vi "Voigt_Fit_DLL_Test.vi"() -> ()   [LabVIEW 2020]
doc: "Test the operation of the Lorentzian Model Fit DLL inside LabVIEW\n\nThe code should do the following\n1. read in a data file containing measured LLM data [freq (MHz), spctrm (dBm)]\n1a. select a subset of the data from some subset of the freq range (optional)\n2. provide initial guesses for the fitting parameters\n3. call the function Lorentz_Fit from the DLL\n\nR. Sheehan 9 - 11 - 2021"
uses:
  <vilib>/Utility/file.llb/Read Delimited Spreadsheet (DBL).vi
panel:
  out "Lor_gof":dbl[](array[numeric])=[3199.0, 1.0009386733416772, 0.954874518705434, 0.4817149539059473]
  out "L_pars":dbl[](array[numeric])=[0.7072584069399376, 80.0, 1.7560129064005117]
  out "Voigt LLM / MHz":dbl
  in  "Freqs":T1={"Ffitlo / MHz"=70.0, "Fcentre / MHz"=80.0, "Ffithi / MHz"=90.0, "Lor HWHM / MHz"=2.6187499999999915, "Peak Est / nW"=0.0, "Gau stdev / MHz "=2.6187499999999915}
  in  "Fcentre / MHz":dbl=80.0
  out "gof_stats":dbl[](array[numeric])=[4799.0, 1.000625521267723, 0.9428903903200956, 0.4850704566774246]
  out "V_pars":dbl[](array[numeric])=[2.3238013033110674, 80.0, 1.3781481716459836]
  out "FileName":path=path "C:/Users/robertsheehan/Programming/LabVIEW/Textronix_RSA2203A/Sample_Data/Smpl_LLM_1.txt"
  in  "Ffithi / MHz":dbl=95.0
  in  "Ffitlo / MHz":dbl=65.0
  out "Fmax / MHz":dbl=80.19375
  out "LLest / MHz":dbl=2.299999999999997
  out "Pmax / nW":dbl=1.4094510581310635e-06
  out "Pmax / dBm":dbl=-58.5095
  out "Flo / MHz":dbl=60.0
  out "Fhi / MHz":dbl=100.0
  out "LLM Output":cluster{"all rows":dbl[], "all rows":dbl[]}[](graph)
  out "TheData":dbl[][](array[numeric])
  # "Amp. Par\n\nAOM Freq / MHz\n\nLor HWHM / MHz\n\nGau Stdev / MHz"
  # "Amp. Par\n\nAOM Freq / MHz\n\nLor HWHM / MHz"
  # "chi^{2} for the fit\n\nchi^{2} / nu\n\nR^{2}\n\nGOF"
  # "chi^{2} for the fit\n\nchi^{2} / nu\n\nR^{2}\n\nGOF"
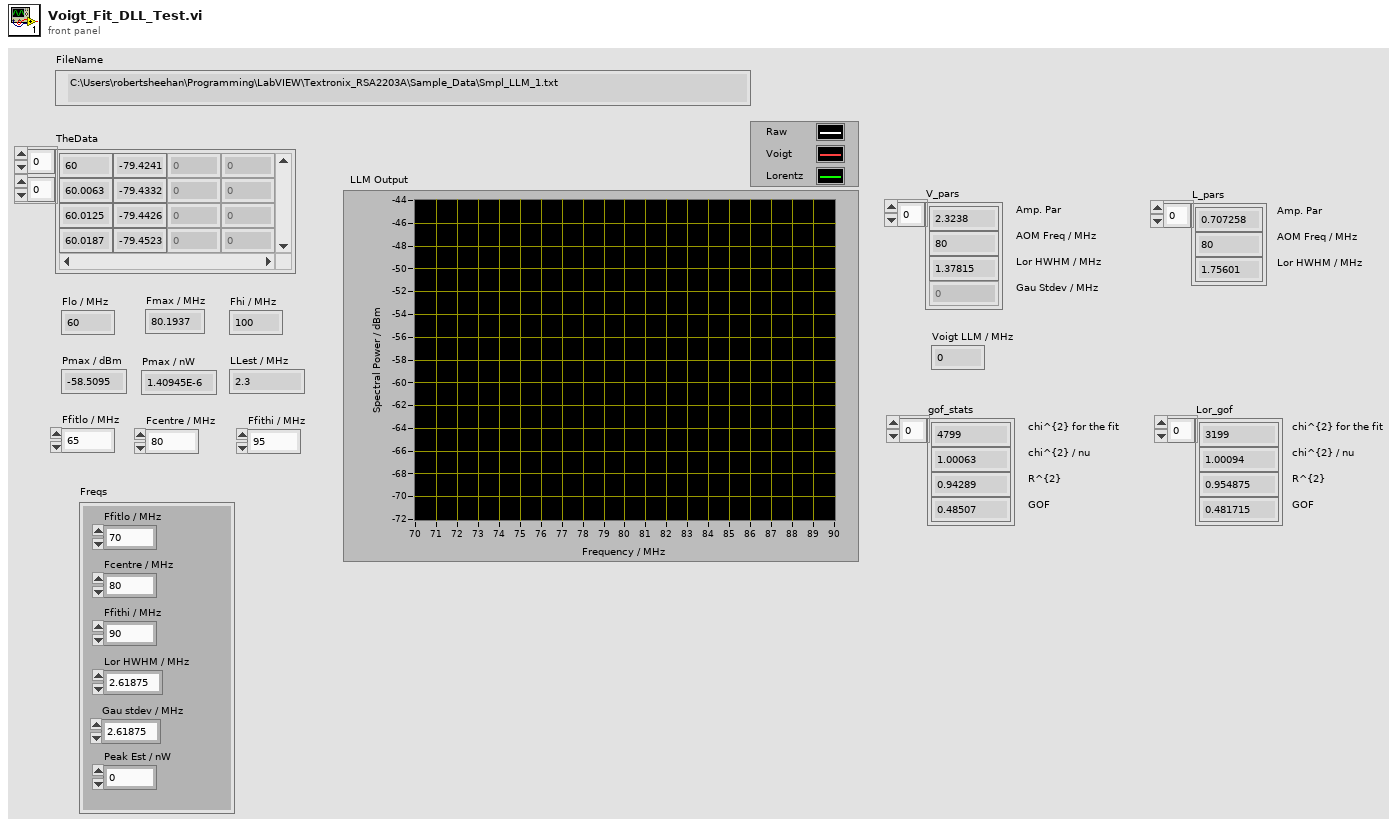
[diagram p1: front panel]
types:
  T1 = cluster{"Ffitlo / MHz":dbl, "Fcentre / MHz":dbl, "Ffithi / MHz":dbl, "Lor HWHM / MHz":dbl, "Peak Est / nW":dbl, "Gau stdev / MHz ":dbl}
  T2 = cluster{"freq_fit_data":dbl[], "spctrm_fit_data":dbl[]}
  T3 = cluster{"freq_fit_data":dbl[], "spctrm_fit_data":dbl[]}[]
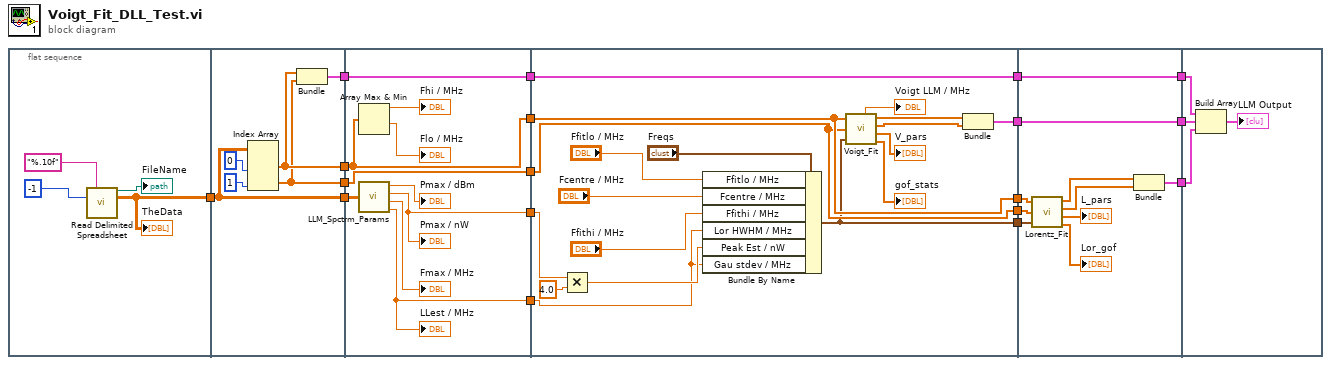
[diagram p0: block diagram]
diagram:
  n1 = flat-sequence {
    tunnel: [w20] -> w18
    tunnel: w18 -> [w26]
    tunnel: [w25] -> w17
    tunnel: [w26] -> w16
    tunnel: [w24] -> w15
    tunnel: [w23] -> w14
    tunnel: w17 -> [w31]
    tunnel: w16 -> [w37]
    tunnel: w15 -> [w30]
    tunnel: w14 -> [w32]
    tunnel: [w33] -> w13
    tunnel: [w32] -> w11
    tunnel: [w31] -> w10
    tunnel: [w30] -> w9
    tunnel: [w29] -> w8
    tunnel: w13 -> [w44]
    tunnel: [w54] -> w12
    tunnel: w11 -> [w54]
    tunnel: w10 -> [w42]
    tunnel: w9 -> [w41]
    tunnel: w8 -> [w51]
    tunnel: [w42] -> w7
    tunnel: [w41] -> w6
    tunnel: [w40] -> w5
    tunnel: [w39] -> w4
    tunnel: w12 -> [w60]
    tunnel: w7 -> [w63]
    tunnel: w6 -> [w62]
    tunnel: w5 -> [w61]
    tunnel: [w60] -> w3
    tunnel: [w59] -> w2
    tunnel: w4 -> [w59]
    tunnel: [w58] -> w1
    tunnel: w3 -> [w70]
    tunnel: w2 -> [w69]
    tunnel: w1 -> [w68]
    frame #0 {
      n2 = call-poly <vilib>:"Read Delimited Spreadsheet.vi"("format (%.3f)"="%.10f", "number of rows (all:-1)"=-1) -> ("new file path (Not A Path if cancelled)"=→"FileName":path, "all rows"=w20:dbl[][])  [unwired: 8 in, 4 out]
      "TheData" <- w20
    }
    frame #1 {
      n3 = Index Array(array=w26, index (col) #1=0 ("disabled index (col)"), index (col) #2=1 ("index (col)")) -> (element #1=w25:dbl[], element #2=w24:dbl[])  [unwired: 2 in]
      n4 = Bundle("all rows"=w25, "all rows"=w24) -> (w23:cluster{"all rows":dbl[], "all rows":dbl[]})  [unwired: 1 in]
    }
    frame #2 {
      n5 = Array Max & Min(array=w31) -> (max value=→"Fhi / MHz":dbl, min value=→"Flo / MHz":dbl)  [unwired: 2 out]
      n6 = call "LLM_Spctrm_Params.vi"("Data"=w37) -> ("Pmax / dBm"=→"Pmax / dBm":dbl, "Pmax / nW"=w29:dbl, "Fmax / MHz"=→"Fmax / MHz":dbl, "LL / MHz"=w33:dbl)
      "Pmax / nW" <- w29
      "LLest / MHz" <- w33
    }
    frame #3 {
      n7 = Multiply(x=w51, y=4.0) -> (x*y=w45:dbl)
      n8 = Bundle By Name(cluster="Freqs", "Ffitlo / MHz"="Ffitlo / MHz", "Fcentre / MHz"="Fcentre / MHz", "Ffithi / MHz"="Ffithi / MHz", "Lor HWHM / MHz"=w44, "Peak Est / nW"=w45, "Gau stdev / MHz"=w44) -> (w40:T1)
      n9 = call "Voigt_Fit.vi"("Freq_Data"=w42, "Scptrm_Data"=w41, "Freqs"=w40) -> ("freq_fit_data"=w53:dbl[], "spctrm_fit_data"=w52:dbl[], "a_pars"=→"V_pars":dbl[], "gof_stats"=→"gof_stats":dbl[], "Voigt LLM"=→"Voigt LLM / MHz":dbl)
      n10 = Bundle("freq_fit_data"=w53, "spctrm_fit_data"=w52) -> (w39:T2)  [unwired: 1 in]
    }
    frame #4 {
      n11 = call "Lorentz_Fit.vi"("Freq_Data"=w63, "Scptrm_Data"=w62, "Freqs"=w61) -> ("freq_fit_data"=w66:dbl[], "spctrm_fit_data"=w65:dbl[], "a_pars"=→"L_pars":dbl[], "gof_stats"=→"Lor_gof":dbl[])
      n12 = Bundle("freq_fit_data"=w66, "spctrm_fit_data"=w65) -> (w58:T2)  [unwired: 1 in]
    }
    frame #5 {
      n13 = Build Array(w70, w69, w68) -> (→"LLM Output":T3)
    }
  }
